vi "VI, Set Panel Width.vi"(5 "width":i16=20, 6 "error in":errorcluster, 9 "VI ref":refnum<vi>) -> (0 "error out":errorcluster, 3 "VI ref dup":refnum<vi>)   [LabVIEW 2010]
doc: "This function sets a panel width in pixel units by adjusting the right boundary. The panel position is unchanged."
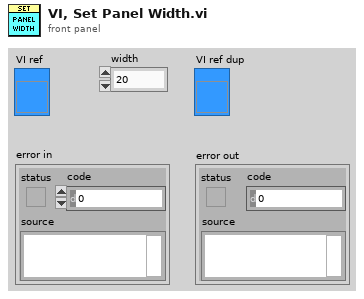
[diagram p1: front panel]
types:
  T1 = typedef "LVRectTypeDef.ctl" = cluster{"left":i16, "top":i16, "right":i16, "bottom":i16}
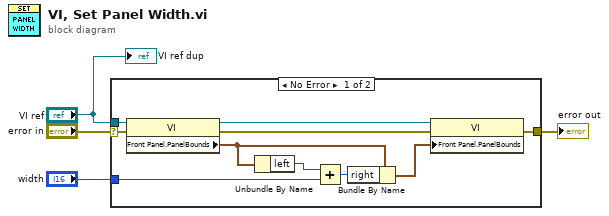
[diagram p0: block diagram]
diagram:
  n1 = case shown="No Error" "error in" {
    selector: "error in" -> [w9 w15]
    tunnel: "VI ref" -> [w13 _]
    tunnel: [w10 w15] -> w4
    tunnel: "width" -> [w5 _]
    frame No Error {
      n2 = property class="VI"(reference=w13, error in=w9) -> (reference out=w7:refnum<vi>, error out=w8:errorcluster, "Front Panel.PanelBounds"=w12:T1)
      n3 = Unbundle By Name(w12) -> ("left"=w6:i16)
      n4 = Add(x=w6, y=w5) -> (x+y=w11:i16)
      n5 = Bundle By Name(cluster=w12, "right"=w11) -> (w14:T1)
      n6 = property class="VI"(reference=w7, error in=w8, "Front Panel.PanelBounds"=w14) -> (error out=w10:errorcluster)  [unwired: 1 out]
    }
    frame Error {
    }
  }
  "error out" <- w4
  "VI ref dup" <- "VI ref"
